vi "Save Image by User.vi"(8 "error in (no error)":errorcluster, 11 "IMAQ Display in":refnum<class "HIJ Vision Camera App.lvclass">) -> (0 "error out":errorcluster, 3 "IMAQ Display out":refnum<class "HIJ Vision Camera App.lvclass">)   [LabVIEW 2020, in "HIJ Vision Camera App.lvlib" / "HIJ Vision Camera App.lvclass"]
doc: "Speichert das Kamerabild in PNG Format und ruft Generate Report auf. Wenn Flag \"Time in Filename\" gesetzt ist, wird ein Zeitstempel dem Dateinamen angehängt."
uses:
  HIJ Vision Camera App.lvclass
  C:/Users/AlexK/work/LabVIEW Programme/POLARIS CAM Log Abw und E/Submodules/HIJ Vision/Application Base Actors/HIJ Vision Application/HIJ Vision Application/HIJ Vision Application.lvclass
  HIJ Vision Application/HIJ Vision Application/HIJ Vision Application.lvclass/HIJ Vision Application.ctl
  <vilib>/ActorFramework/Message Enqueuer/Message Enqueuer.lvclass/Message Enqueuer.ctl
  HIJ Vision Application/HIJ Vision Application/Read Display Enq.vi
  <vilib>/ActorFramework/Message Enqueuer/Enqueue.vi
  Display Actors/HIJ Vision Display/HIJ Vision Display Messages/Save Image Msg/Save Image Msg.lvclass
  C:/Program Files (x86)/National Instruments/LabVIEW 2020/vi.lib/ActorFramework/Message/Message.lvclass
  <vilib>/ActorFramework/Message Priority Queue/Priority Enqueue.vi
  <vilib>/ActorFramework/Message Enqueuer/Message Enqueuer.lvclass
  HIJ Vision Camera App.lvclass/HIJ Vision Camera App.ctl
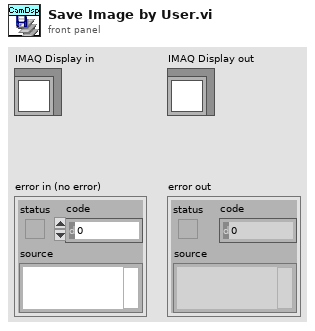
[diagram p1: front panel]
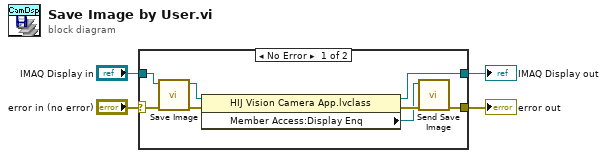
[diagram p0: block diagram]
diagram:
  n1 = case shown="No Error" "error in (no error)" {
    selector: "error in (no error)" -> [w6 w14]
    tunnel: [w9 w14] -> w3
    tunnel: [w8 w13] -> w1
    tunnel: "IMAQ Display in" -> [w7 w13]
    frame No Error {
      n2 = call-dynamic "Save Image.vi"("error in (no error)"=w6, "IMAQ Display in"=w7) -> ("error out"=w11:errorcluster, "IMAQ Display out"=w12:refnum<class "HIJ Vision Camera App.lvclass">)  [unwired: 8 in]
      n3 = property class="HIJ Vision Camera App.lvclass"(reference=w12, error in=w11) -> (reference out=w8:refnum<class "HIJ Vision Camera App.lvclass">, error out=w10:errorcluster, "Member Access:Display Enq"=w5:refnum<class "Message Enqueuer.lvclass">)
      n4 = call "Send Save Image.vi"("error in (no error)"=w10, "Message Enqueuer"=w5) -> ("error out"=w9:errorcluster)  [unwired: 8 in, 1 out]
    }
    frame Error {
    }
  }
  "error out" <- w3
  "IMAQ Display out" <- w1
